vi "Autotrace.vi"() -> (2 "Center Position":dbl[](array[numeric])=[100.0, 100.0, 100.0], 3 "Final Count Rate":dbl format="%#.10g")   [LabVIEW 2020]
uses:
  Global Parameters.vi
  Global Parameter/NV Global.vi
  labview_control/LaoJi/NI CTR/NI DAQ Counter.lvlib
  Labview Library/Libraries/ASG8100CY/ASG8100CY.lvlib
panel:
  in  "Sample Rate (Hz)":dbl=50.0
  out "AutoTrace Data":dbl[][](array[numeric])
  in  "name":string="NV_1.17_"
  in  "save?":bool
  in  "Tab Control":T1(tab)
  in  "Stop":bool
  out "Start Point":dbl[](array[numeric])
  in  "Diameter xy":dbl=4.0
  in  "No. of Points":i32=50
  in  "move distance max":dbl=0.5
  in  "Diameter z":dbl=8.0
  out "X Indicator":bool
  out "Y Indicator":bool
  out "Z Indicator":bool
  out "Y":cluster{dbl[], "Best Gaussian Fit":dbl[]}[](graph)=[{[28.587433264887064, 28.667433264887062, 28.747433264887064, 28.827433264887063, 28.907433264887064, 28.987433264887063, 29.067433264887065, 29.147433264887063, 29.227433264887065, 29.307433264887063, 29.387433264887065, 29.467433264887063, 29.547433264887065, 29.627433264887063, 29.707433264887065, 29.787433264887063, 29.867433264887065, 29.947433264887064, 30.027433264887065, 30.107433264887064, 30.187433264887066, 30.267433264887064, 30.347433264887066, 30.427433264887064, 30.507433264887062, 30.587433264887064, 30.667433264887066, 30.747433264887064, 30.827433264887063, 30.907433264887064, 30.987433264887063, 31.067433264887065, 31.147433264887063, 31.227433264887065, 31.307433264887063, 31.387433264887065, 31.467433264887063, 31.547433264887065, 31.627433264887063, 31.707433264887065, 31.787433264887063, 31.867433264887065, 31.947433264887064, 32.027433264887065, 32.107433264887064, 32.18743326488706, 32.26743326488707, 32.347433264887066, 32.427433264887064, 32.50743326488706], "Best Gaussian Fit"=[82695.7939382761, 93035.93239563631, 104208.75707394363, 116210.11359683966, 129023.80448201254, 142620.50495842184, 156956.86080825518, 171974.8132803884, 187601.19363183164, 203747.62553370168, 220310.76741984417, 237172.9189336669, 254203.00610454116, 271257.94900932355, 288184.403780577, 304820.8583173002, 321000.0484018995, 336551.6486337933, 351305.1811783909, 365093.0753155868, 377753.80263689667, 389135.00690826605, 399096.5444274202, 407513.3503978308, 414278.0495345521, 419303.2347992863, 422523.34668930905, 423896.09660369105, 423403.39108770975, 421051.7287169694, 416872.0574510246, 410919.09683369054, 403270.14579218073, 394023.4123464537, 383295.9156795657, 371221.0232029976, 357945.6950340998, 343627.5153542803, 328431.5942305132, 312527.42458537646, 296085.7771505447, 279275.71161830187, 262261.775109772, 245201.44989429894, 228242.90147961042, 211523.06625001764, 195166.10528265772, 179282.23833600763, 163966.95976739613, 149300.62673344553]}, {[28.587433264887064, 28.667433264887062, 28.747433264887064, 28.827433264887063, 28.907433264887064, 28.987433264887063, 29.067433264887065, 29.147433264887063, 29.227433264887065, 29.307433264887063, 29.387433264887065, 29.467433264887063, 29.547433264887065, 29.627433264887063, 29.707433264887065, 29.787433264887063, 29.867433264887065, 29.947433264887064, 30.027433264887065, 30.107433264887064, 30.187433264887066, 30.267433264887064, 30.347433264887066, 30.427433264887064, 30.507433264887062, 30.587433264887064, 30.667433264887066, 30.747433264887064, 30.827433264887063, 30.907433264887064, 30.987433264887063, 31.067433264887065, 31.147433264887063, 31.227433264887065, 31.307433264887063, 31.387433264887065, 31.467433264887063, 31.547433264887065, 31.627433264887063, 31.707433264887065, 31.787433264887063, 31.867433264887065, 31.947433264887064, 32.027433264887065, 32.107433264887064, 32.18743326488706, 32.26743326488707, 32.347433264887066, 32.427433264887064, 32.50743326488706], "Best Gaussian Fit"=[0.0, 0.0, 0.0, 0.0, 0.0, 206291.54274517627, 210191.98673408732, 213652.8090545292, 210992.13509832733, 225995.6712662076, 229171.96204752172, 235716.96444444387, 260374.20344517086, 269183.87857142655, 282045.01726815425, 300870.52845503774, 336014.8514509855, 352432.5725864057, 368076.08672803076, 394901.02495494834, 414560.21447765, 432489.6705639836, 433552.6213811527, 438455.5715313964, 455299.529286137, 456372.0008292065, 459809.01578123606, 444017.0537733845, 438784.5826197389, 420773.64736858197, 379644.37848563184, 369423.66261220514, 344908.61083223054, 340345.2079602573, 322023.16098694917, 308115.01870457915, 290468.51555417373, 283489.69824613957, 283962.05635919375, 283721.7296458335, 283917.8453180592, 277165.3062343066, 272160.0475794274, 261937.72177790813, 260232.55700557673, 258499.65012753732, 247613.77779795573, 246263.40366328714, 240502.41945111495, 243778.22832663747]}]
  out "X":cluster{dbl[], "Best Gaussian Fit":dbl[]}[](graph)=[{[30.618585858585853, 30.69858585858585, 30.778585858585853, 30.85858585858585, 30.938585858585853, 31.01858585858585, 31.098585858585853, 31.17858585858585, 31.258585858585853, 31.33858585858585, 31.418585858585853, 31.49858585858585, 31.578585858585853, 31.65858585858585, 31.738585858585854, 31.818585858585852, 31.898585858585854, 31.978585858585852, 32.05858585858585, 32.138585858585856, 32.218585858585854, 32.29858585858585, 32.37858585858585, 32.458585858585856, 32.538585858585854, 32.61858585858585, 32.69858585858585, 32.778585858585856, 32.858585858585855, 32.93858585858585, 33.01858585858585, 33.09858585858585, 33.178585858585855, 33.25858585858585, 33.33858585858585, 33.41858585858585, 33.498585858585855, 33.57858585858585, 33.65858585858585, 33.73858585858585, 33.818585858585855, 33.898585858585854, 33.97858585858585, 34.05858585858585, 34.138585858585856, 34.218585858585854, 34.29858585858585, 34.37858585858585, 34.45858585858585, 34.538585858585854], "Best Gaussian Fit"=[199622.7652092626, 213700.13322189654, 227947.77524969875, 242271.18422272106, 256568.8961464526, 270733.556571258, 284653.1608456071, 298212.4509139653, 311294.44639794744, 323782.08305597847, 335559.92762615264, 346515.93468145275, 356543.20861001866, 365541.7322943554, 373420.0235902078, 380096.6813503637, 385501.7845142223, 389578.11066303233, 392282.1443552326, 393584.85039918293, 393472.1928493558, 391945.38675389026, 389020.87633961934, 384730.040182248, 379118.63075326587, 372245.9623411023, 364183.8675010448, 355015.44770309766, 344833.6485509264, 333739.6937011037, 321841.41431907495, 309251.5125047676, 296085.79758573393, 282461.43352867546, 268495.2340192452, 254302.03909833776, 239993.20374368748, 225675.2245959362, 211448.52631291925, 197406.42396979578, 183634.2726835259, 170208.81040218376, 157197.6947260679, 144659.22986625435, 132642.27552394307, 121186.32569384929, 110321.74223363581, 100070.12554876537, 90444.80294075941, 81451.41405397304]}, {[30.618585858585853, 30.69858585858585, 30.778585858585853, 30.85858585858585, 30.938585858585853, 31.01858585858585, 31.098585858585853, 31.17858585858585, 31.258585858585853, 31.33858585858585, 31.418585858585853, 31.49858585858585, 31.578585858585853, 31.65858585858585, 31.738585858585854, 31.818585858585852, 31.898585858585854, 31.978585858585852, 32.05858585858585, 32.138585858585856, 32.218585858585854, 32.29858585858585, 32.37858585858585, 32.458585858585856, 32.538585858585854, 32.61858585858585, 32.69858585858585, 32.778585858585856, 32.858585858585855, 32.93858585858585, 33.01858585858585, 33.09858585858585, 33.178585858585855, 33.25858585858585, 33.33858585858585, 33.41858585858585, 33.498585858585855, 33.57858585858585, 33.65858585858585, 33.73858585858585, 33.818585858585855, 33.898585858585854, 33.97858585858585, 34.05858585858585, 34.138585858585856, 34.218585858585854, 34.29858585858585, 34.37858585858585, 34.45858585858585, 34.538585858585854], "Best Gaussian Fit"=[0.0, 0.0, 0.0, 0.0, 0.0, 427244.8722271027, 437596.2068010136, 438557.34292178537, 447522.7808637517, 450272.5610295557, 462861.06273628754, 465668.3899037813, 460005.58720065054, 456337.9991536631, 449257.817837283, 448342.5759616434, 436186.2288725173, 430644.30916723004, 419807.75032678, 400558.9430741828, 384481.8022328452, 372598.71866850153, 355275.13386246277, 342864.4763392376, 318625.43663690117, 305968.09319236135, 295158.16662579577, 280150.94194027554, 263182.40619435295, 256594.04351134866, 253517.6315882785, 246929.03603153766, 242208.0360085657, 228934.00480565085, 225579.11596168345, 218747.91014951197, 215025.77963564653, 207010.84932462528, 210830.96445404616, 206259.81180164526, 204225.92522338819, 210423.6634213615, 203684.5686192836, 209968.62289134995, 204533.09352025428, 206559.33826787924, 203394.15591947164, 207928.7397448016, 205453.0602229333, 201667.86139781526]}]
  out "Z":cluster{dbl[], "Best Gaussian Fit":dbl[]}[](graph)=[{[47.76000000000001, 47.92000000000001, 48.08000000000001, 48.24000000000001, 48.40000000000001, 48.56000000000001, 48.72000000000001, 48.88000000000001, 49.04000000000001, 49.20000000000001, 49.360000000000014, 49.52000000000001, 49.680000000000014, 49.84000000000001, 50.000000000000014, 50.16000000000001, 50.320000000000014, 50.48000000000001, 50.640000000000015, 50.80000000000001, 50.960000000000015, 51.12000000000001, 51.280000000000015, 51.44000000000001, 51.60000000000001, 51.76000000000001, 51.920000000000016, 52.08000000000001, 52.24000000000001, 52.40000000000001, 52.56000000000001, 52.72000000000001, 52.88000000000001, 53.04000000000001, 53.20000000000001, 53.360000000000014, 53.52000000000001, 53.680000000000014, 53.84000000000001, 54.000000000000014, 54.16000000000001, 54.320000000000014, 54.48000000000001, 54.640000000000015, 54.80000000000001, 54.960000000000015, 55.12000000000001, 55.280000000000015, 55.44000000000001, 55.60000000000001], "Best Gaussian Fit"=[209099.73307391262, 218503.14461197148, 229355.6959593358, 241719.88156101448, 255620.83493327926, 271037.87859240867, 287896.9703361263, 306064.70466487855, 325344.52746696095, 345475.76446683565, 366135.9454640973, 386946.72907660797, 407483.5051154103, 427288.4889323076, 445886.84477118263, 462805.10789012676, 477590.94406552694, 489833.11476363277, 499180.42722509126, 505358.4545023384, 508182.9157852256, 507568.80692190514, 503534.6499186207, 496201.56499610166, 485787.2300702261, 472595.14800389623, 456999.9599731276, 439429.79620230943, 420346.82253882475, 400227.211264221, 379541.735522225, 358738.06678508525, 338225.66015664616, 318363.86532424996, 299453.6271605823, 281732.8651797201, 265375.36869575386, 250492.83345338725, 237139.50851200195, 225318.8254649993, 214991.345461141, 206083.37725441426, 198495.6818046096, 192111.77343650526, 186805.44102964734, 182447.23253688062, 178909.76143960972, 176071.79614687152, 173821.17726175574, 172056.67029302815]}, {[47.76000000000001, 47.92000000000001, 48.08000000000001, 48.24000000000001, 48.40000000000001, 48.56000000000001, 48.72000000000001, 48.88000000000001, 49.04000000000001, 49.20000000000001, 49.360000000000014, 49.52000000000001, 49.680000000000014, 49.84000000000001, 50.000000000000014, 50.16000000000001, 50.320000000000014, 50.48000000000001, 50.640000000000015, 50.80000000000001, 50.960000000000015, 51.12000000000001, 51.280000000000015, 51.44000000000001, 51.60000000000001, 51.76000000000001, 51.920000000000016, 52.08000000000001, 52.24000000000001, 52.40000000000001, 52.56000000000001, 52.72000000000001, 52.88000000000001, 53.04000000000001, 53.20000000000001, 53.360000000000014, 53.52000000000001, 53.680000000000014, 53.84000000000001, 54.000000000000014, 54.16000000000001, 54.320000000000014, 54.48000000000001, 54.640000000000015, 54.80000000000001, 54.960000000000015, 55.12000000000001, 55.280000000000015, 55.44000000000001, 55.60000000000001], "Best Gaussian Fit"=[0.0, 0.0, 0.0, 0.0, 0.0, 393271.00128946366, 407480.41678200994, 410814.7341749502, 426521.3026883778, 430066.65285827825, 443370.58597368945, 459367.2602933661, 461823.6110592089, 461604.39051720646, 457673.8141300071, 471897.3992822233, 475269.15246727964, 494259.5933463088, 489318.74382746057, 485038.7774016339, 492418.5246702464, 492340.1061251857, 496258.93171883747, 470118.45592524635, 447906.92402490036, 444693.88179068966, 425436.1282296754, 414968.0652258372, 401415.1316234149, 383381.7960970132, 371446.81388909504, 349417.72365313204, 332184.68010942376, 320808.8198801387, 312936.86398166575, 298427.2357123923, 292511.01335288194, 279437.24177576846, 273899.5635723089, 263004.1825411595, 257646.11261281034, 247225.51752630447, 245565.812568203, 241101.30046311184, 235636.8265278222, 232213.79944477836, 231398.6192754935, 224071.13931402928, 221070.99157966094, 218976.58246620942]}]
  out "Z Line Position":dbl[](array[numeric])=[-4.0, -3.84, -3.68, -3.52, -3.36, -3.2, -3.04, -2.88, -2.7199999999999998, -2.56, -2.4, -2.24, -2.08, -1.92, -1.7599999999999998, -1.6, -1.44, -1.2799999999999998, -1.12, -0.96, -0.7999999999999998, -0.6400000000000001, -0.48, -0.31999999999999984, -0.16000000000000014, 0.0, 0.16000000000000014, 0.3200000000000003, 0.4800000000000004, 0.6399999999999997, 0.7999999999999998, 0.96, 1.12, 1.2800000000000002, 1.4400000000000004, 1.6000000000000005, 1.7599999999999998, 1.92, 2.08, 2.24, 2.4000000000000004, 2.5600000000000005, 2.7199999999999998, 2.88, 3.04, 3.2, 3.3600000000000003, 3.5200000000000005, 3.6799999999999997, 3.84, 4.0]
  out "X Line Position":dbl[](array[numeric])=[-2.0, -1.92, -1.84, -1.76, -1.68, -1.6, -1.52, -1.44, -1.3599999999999999, -1.28, -1.2, -1.12, -1.04, -0.96, -0.8799999999999999, -0.8, -0.72, -0.6399999999999999, -0.56, -0.48, -0.3999999999999999, -0.32000000000000006, -0.24, -0.15999999999999992, -0.08000000000000007, 0.0, 0.08000000000000007, 0.16000000000000014, 0.2400000000000002, 0.31999999999999984, 0.3999999999999999, 0.48, 0.56, 0.6400000000000001, 0.7200000000000002, 0.8000000000000003, 0.8799999999999999, 0.96, 1.04, 1.12, 1.2000000000000002, 1.2800000000000002, 1.3599999999999999, 1.44, 1.52, 1.6, 1.6800000000000002, 1.7600000000000002, 1.8399999999999999, 1.92, 2.0]
  out "Y line Position":dbl[](array[numeric])=[-2.0, -1.92, -1.84, -1.76, -1.68, -1.6, -1.52, -1.44, -1.3599999999999999, -1.28, -1.2, -1.12, -1.04, -0.96, -0.8799999999999999, -0.8, -0.72, -0.6399999999999999, -0.56, -0.48, -0.3999999999999999, -0.32000000000000006, -0.24, -0.15999999999999992, -0.08000000000000007, 0.0, 0.08000000000000007, 0.16000000000000014, 0.2400000000000002, 0.31999999999999984, 0.3999999999999999, 0.48, 0.56, 0.6400000000000001, 0.7200000000000002, 0.8000000000000003, 0.8799999999999999, 0.96, 1.04, 1.12, 1.2000000000000002, 1.2800000000000002, 1.3599999999999999, 1.44, 1.52, 1.6, 1.6800000000000002, 1.7600000000000002, 1.8399999999999999, 1.92, 2.0]
  in  "Limit":T2={"width threshold -"=0.05, "width threshold +"=6.0, "counts threshold"=15000.0}
  out "NV or not?":bool
  out "Laser On":bool=TRUE
  out "Positioner\nerror":errorcluster
  in  "AutoTrace \nData base path":path=path "I:/AutoTrace"
  # "Counter Settings"
  # "Clock Settings"
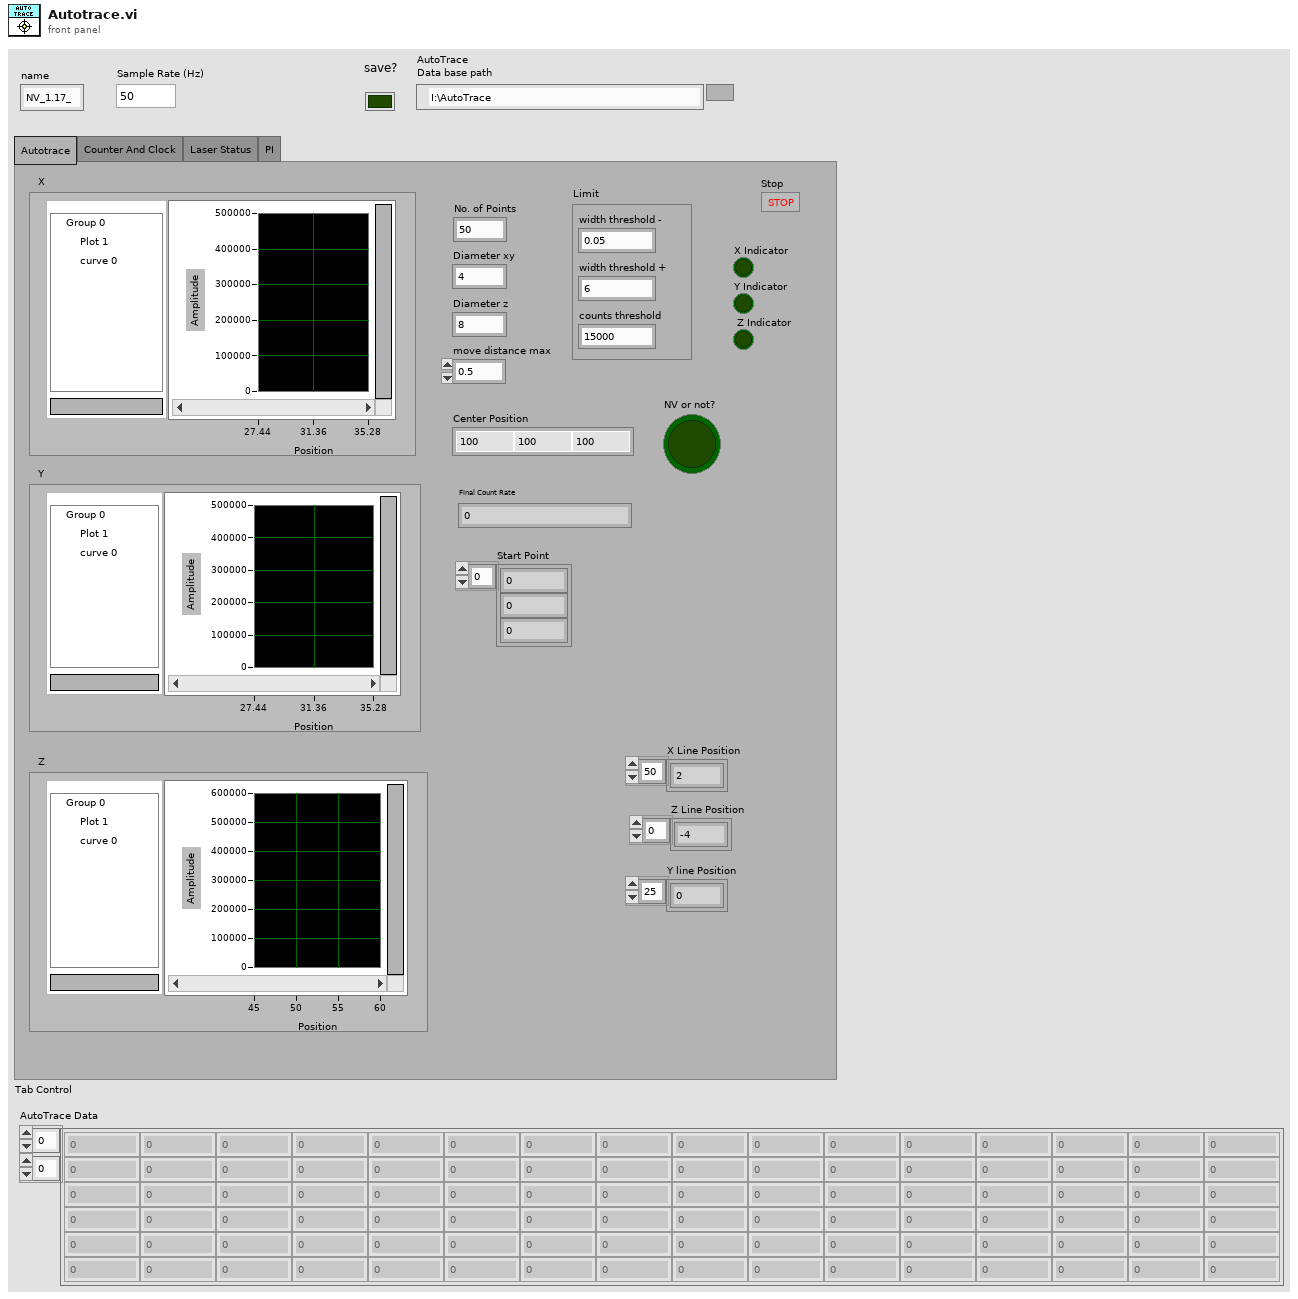
[diagram p1: front panel]
types:
  T1 = enum32{"Autotrace", "Counter And Clock", "Laser Status", "PI"}
  T2 = cluster{"width threshold -":dbl, "width threshold +":dbl, "counts threshold":dbl}
  T3 = typedef "imagedata.ctl" = cluster{"image type":i32, "image depth":i32, "image":u8[], "mask":u8[], "colors":u32[], "Rectangle":cluster{"left":i16, "top":i16, "right":i16, "bottom":i16}}
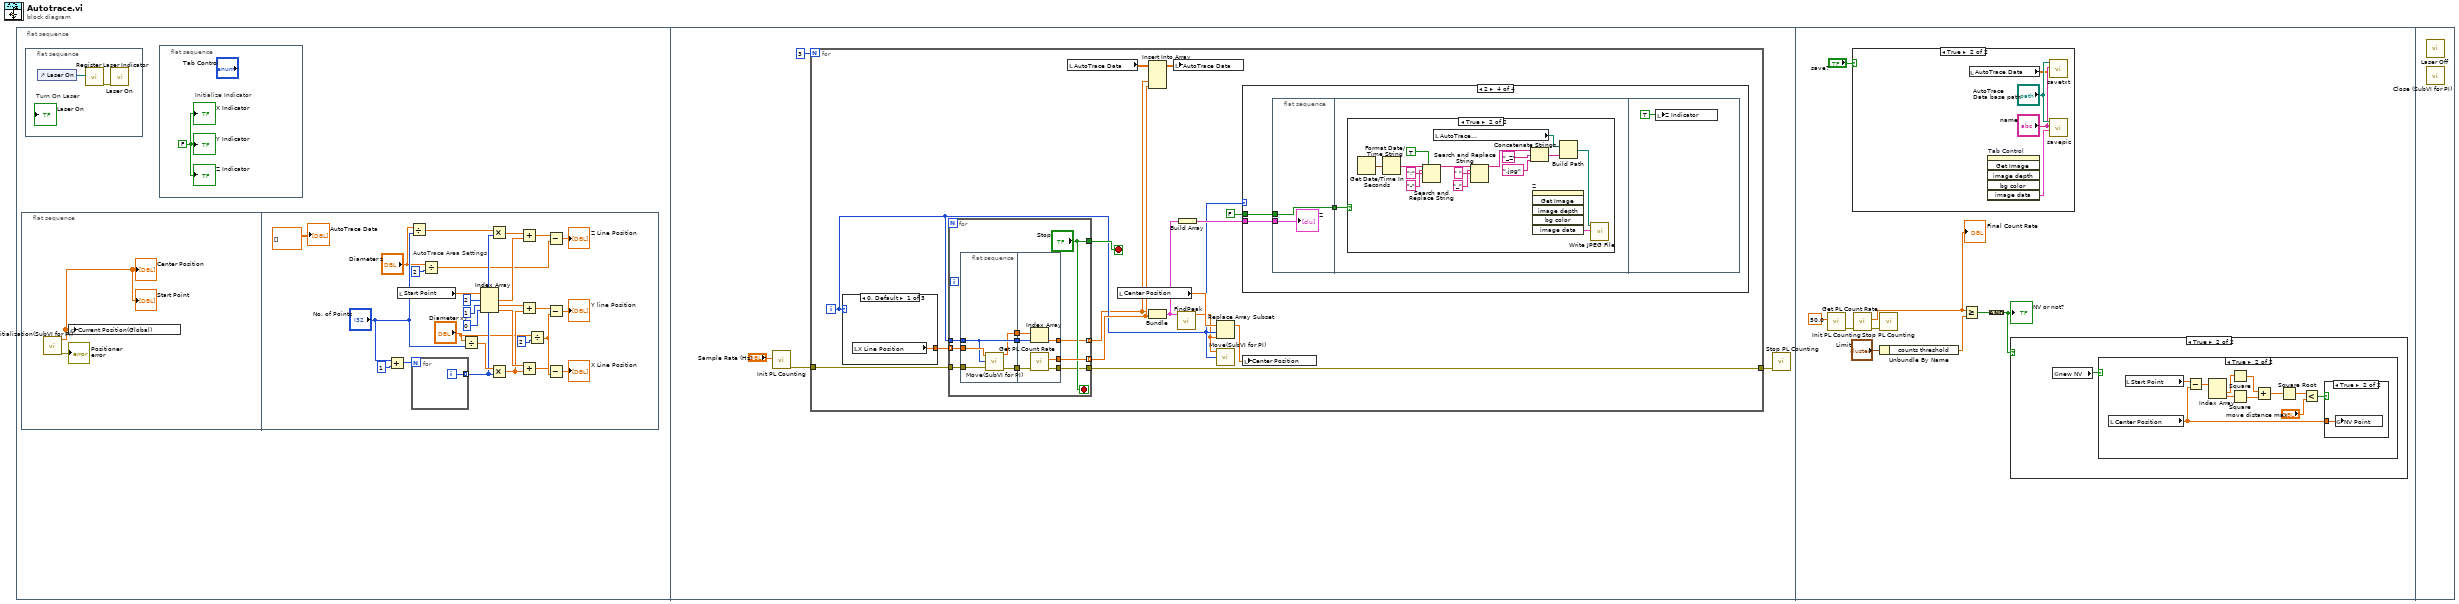
[diagram p0: block diagram]
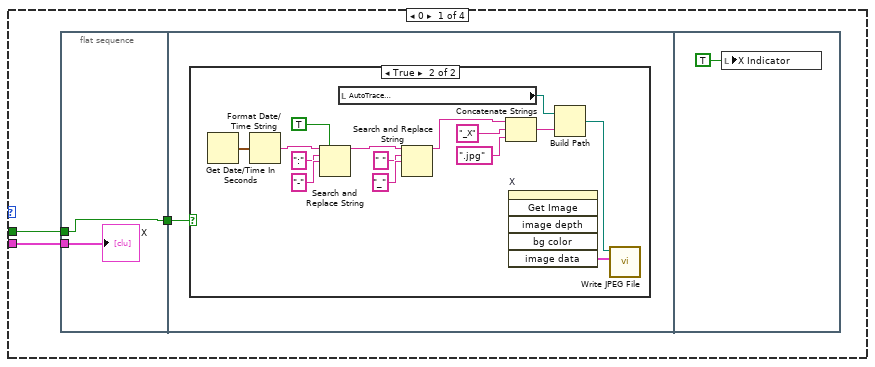
[diagram p2: hidden frame]
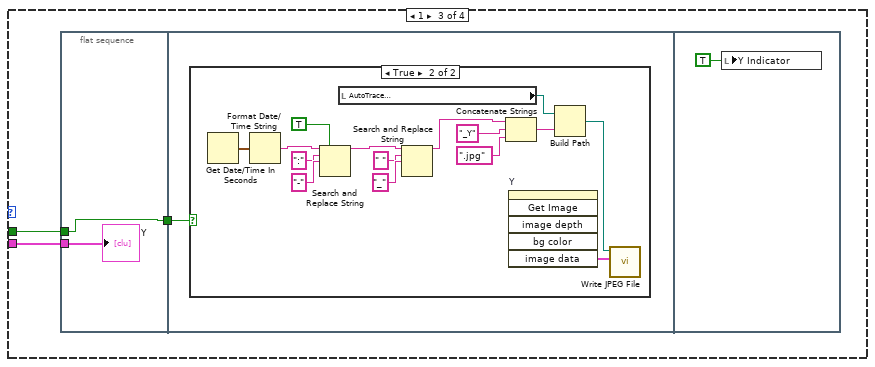
[diagram p5: hidden frame]
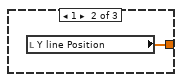
[diagram p8: hidden frame]
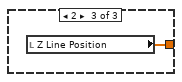
[diagram p9: hidden frame]
diagram:
  n1 = flat-sequence {
    frame #0 {
      n2 = flat-sequence {
        frame #0 {
          n3 = call "Initialization(SubVI for PI).vi"() -> ("error out"=→"Positioner\nerror":errorcluster, "Position"=w4:dbl[])  [unwired: 10 in]
          "Start Point" <- w4
          "Center Position" <- w4
          n4 = global write "Global Parameters.vi" "Current Position(Global)"(w4) -> ()
        }
        frame #1 {
          # "AutoTrace Area Settings"
          n5 = Add(x="No. of Points", y=1) -> (x+y=w32:i32)
          n6 = local read "Start Point"() -> (w24:dbl[])
          n7 = Divide(x="Diameter z", y="No. of Points") -> (x/y=w28:dbl)
          n8 = for {
            N: w32 -> [_]
            tunnel: [w34] -> w29 mode=indexing
            i -> [w34]
          }
          n9 = Divide(x="Diameter z", y=2) -> (x/y=w16:dbl)
          n10 = Divide(x="Diameter xy", y="No. of Points") -> (x/y=w30:dbl)
          n11 = Index Array(array=w24, index #1=2, index #2=1, index #3=0) -> (element #1=w23:dbl, element #2=w21:dbl, element #3=w20:dbl)
          n12 = Multiply(x=w28, y=w29) -> (x*y=w22:dbl[])
          n13 = Multiply(x=w30, y=w29) -> (x*y=w19:dbl[])
          n14 = Add(x=w22, y=w23) -> (x+y=w18:dbl[])
          n15 = Add(x=w21, y=w19) -> (x+y=w11:dbl[])
          n16 = Add(x=w20, y=w19) -> (x+y=w8:dbl[])
          n17 = Divide(x="Diameter xy", y=2) -> (x/y=w9:dbl)
          n18 = Subtract(x=w18, y=w16) -> (x-y=→"Z Line Position":dbl[])
          n19 = Subtract(x=w11, y=w9) -> (x-y=→"Y line Position":dbl[])
          n20 = Subtract(x=w8, y=w9) -> (x-y=→"X Line Position":dbl[])
          "AutoTrace Data" <- dbl[][] [] ("AutoTrace Data")
        }
      }
      n21 = flat-sequence {
        frame #0 {
          # "Turn On Laser"
          n22 = control-ref of="Laser On"() -> (w3:refnum<vi>)
          n23 = call "Register Laser Indicator.vi"("Laser Indicator Ref"=w3) -> ("error out"=w2:errorcluster)  [unwired: 10 in]
          n24 = call "Laser On.vi"("error in"=w2) -> ()  [unwired: 10 in, 1 out]
        }
      }
      n25 = flat-sequence {
        frame #0 {
          w1 = FALSE
          # "Initialize Indicator"
          "X Indicator" <- w1
          "Y Indicator" <- w1
          "Z Indicator" <- w1
        }
      }
    }
    frame #1 {
      n26 = call "Init PL Counting.vi"("Sample Rate (Hz)"="Sample Rate (Hz)") -> ("error out"=w36:errorcluster)  [unwired: 10 in]
      n27 = for {
        N: 3 -> [_]
        tunnel: w36 -> [w44]
        tunnel: [w43] -> w35
        i -> [w42]
        stop <- w51 stop-if-true
        n28 = case shown="0, Default" w42 {
          tunnel: [w120 w121 w122] -> w40
          frame 0, Default {
            n29 = local read "X Line Position"() -> (w120:dbl[])
          }
          frame 1 {
            n30 = local read "Y line Position"() -> (w121:dbl[])
          }
          frame 2 {
            n31 = local read "Z Line Position"() -> (w122:dbl[])
          }
        }
        n32 = for {
          tunnel: w40 -> [w132] mode=indexing
          tunnel: w42 -> [w131]
          tunnel: [w130] -> w46 mode=indexing
          tunnel: ["Stop"] -> w51
          tunnel: w44 -> [w128]
          tunnel: [w126] -> w43
          tunnel: [w123] -> w39 mode=indexing
          stop <- "Stop" stop-if-true
          n33 = flat-sequence {
            tunnel: w132 -> [w137]
            tunnel: w131 -> [w134]
            tunnel: w128 -> [w136]
            tunnel: [w135] -> w127
            tunnel: [w134] -> w125
            tunnel: [w133] -> w124
            tunnel: [w143] -> w130
            tunnel: w127 -> [w142]
            tunnel: [w141] -> w126
            tunnel: w125 -> [w140]
            tunnel: w124 -> [w139]
            tunnel: [w138] -> w123
            frame #0 {
              n34 = call "Move(SubVI for PI).vi"("Goal"=w137, "index"=w134, "error in"=w136) -> ("Position After Move"=w133:dbl[], "error out"=w135:errorcluster)  [unwired: 3 in]
            }
            frame #1 {
              n35 = Index Array(array=w139, index=w140) -> (element=w138:dbl)
              n36 = call "Get PL Count Rate.vi"("error in (no error)"=w142) -> ("error out"=w141:errorcluster, "Count Rate"=w143:dbl)  [unwired: 8 in, 1 out]
            }
          }
        }
        n37 = local read "AutoTrace Data"() -> (w47:dbl[][])
        n38 = local read "Center Position"() -> (w50:dbl[])
        n39 = Insert Into Array(array=w47, new element #1=w39, new element #2=w46) -> (w48:dbl[][])  [unwired: 2 in]
        n40 = Bundle(w39, w46) -> (w45:cluster{dbl[], dbl[]})  [unwired: 1 in]
        n41 = local write "AutoTrace Data"(w48) -> ()
        n42 = call "FindPeak.vi"("Input XY"=w45) -> ("Peak Position"=w41:dbl)  [unwired: 8 in, 2 out]
        n43 = Build Array(w45) -> (w53:cluster{dbl[], dbl[]}[])
        n44 = Replace Array Subset(array=w50, new element=w41, index=w42) -> (w49:dbl[])
        n45 = call "Move(SubVI for PI).vi"("Goal"=w41, "index"=w42) -> ()  [unwired: 4 in, 2 out]
        n46 = case shown="2" w42 {
          tunnel: w53 -> [w56 _ w78 w100]
          tunnel: FALSE -> [w54 _ w77 w98]
          frame 0 {
            n47 = flat-sequence {
              tunnel: w56 -> [w58]
              tunnel: [w57] -> w55
              tunnel: w54 -> [w57]
              tunnel: w55 -> [w59]
              frame #0 {
                "X" <- w58
              }
              frame #1 {
                n48 = case shown="True" w59 {
                  frame False {
                  }
                  frame True {
                    n49 = Get Date/Time In Seconds() -> (seconds since 1Jan1904=w74:timestamp)
                    n50 = Format Date/Time String(seconds (now)=w74) -> (date/time string=w67:string)  [unwired: 2 out]
                    n51 = Search and Replace String(replace all?=TRUE ("replace all? (F)"), input string=w67, search string=":", replace string="-" ("replace string (\"\")")) -> (result string=w71:string)  [unwired: 1 in, 6 out]
                    n52 = local read "AutoTrace \nData base path"() -> (w60:path)
                    n53 = Search and Replace String(input string=w71, search string=" ", replace string="_" ("replace string (\"\")")) -> (result string=w64:string)  [unwired: 1 in, 7 out]
                    n54 = Concatenate Strings(w64, "_X" ("string"), ".jpg" ("string")) -> (w66:string)
                    n55 = invoke on="X" class="MixedGraph (严格)" method="Get Image"() -> ("image data"=w61:T3)  [unwired: 6 in, 5 out]
                    n56 = Build Path(base path=w60, name or relative path=w66) -> (appended path=w65:path)
                    n57 = call <vilib>:"Write JPEG File.vi"("image data"=w61, "path to JPEG file"=w65) -> ()  [unwired: 1 in, 9 out]
                  }
                }
              }
              frame #2 {
                n58 = local write "X Indicator"(TRUE) -> ()
              }
            }
          }
          frame 3, Default {
          }
          frame 1 {
            n59 = flat-sequence {
              tunnel: w78 -> [w80]
              tunnel: w77 -> [w79]
              tunnel: [w79] -> w76
              tunnel: w76 -> [w81]
              frame #0 {
                "Y" <- w80
              }
              frame #1 {
                n60 = case shown="True" w81 {
                  frame False {
                  }
                  frame True {
                    n61 = Get Date/Time In Seconds() -> (seconds since 1Jan1904=w96:timestamp)
                    n62 = Format Date/Time String(seconds (now)=w96) -> (date/time string=w89:string)  [unwired: 2 out]
                    n63 = Search and Replace String(replace all?=TRUE ("replace all? (F)"), input string=w89, search string=":", replace string="-" ("replace string (\"\")")) -> (result string=w93:string)  [unwired: 1 in, 6 out]
                    n64 = local read "AutoTrace \nData base path"() -> (w86:path)
                    n65 = Search and Replace String(input string=w93, search string=" ", replace string="_" ("replace string (\"\")")) -> (result string=w85:string)  [unwired: 1 in, 7 out]
                    n66 = Concatenate Strings(w85, "_Y" ("string"), ".jpg" ("string")) -> (w88:string)
                    n67 = invoke on="Y" class="MixedGraph (严格)" method="Get Image"() -> ("image data"=w82:T3)  [unwired: 6 in, 5 out]
                    n68 = Build Path(base path=w86, name or relative path=w88) -> (appended path=w87:path)
                    n69 = call <vilib>:"Write JPEG File.vi"("image data"=w82, "path to JPEG file"=w87) -> ()  [unwired: 1 in, 9 out]
                  }
                }
              }
              frame #2 {
                n70 = local write "Y Indicator"(TRUE) -> ()
              }
            }
          }
          frame 2 {
            n71 = flat-sequence {
              tunnel: w100 -> [w102]
              tunnel: [w101] -> w99
              tunnel: w98 -> [w101]
              tunnel: w99 -> [w103]
              frame #0 {
                "Z" <- w102
              }
              frame #1 {
                n72 = case shown="True" w103 {
                  frame False {
                  }
                  frame True {
                    n73 = Get Date/Time In Seconds() -> (seconds since 1Jan1904=w118:timestamp)
                    n74 = Format Date/Time String(seconds (now)=w118) -> (date/time string=w111:string)  [unwired: 2 out]
                    n75 = Search and Replace String(replace all?=TRUE ("replace all? (F)"), input string=w111, search string=":", replace string="-" ("replace string (\"\")")) -> (result string=w115:string)  [unwired: 1 in, 6 out]
                    n76 = local read "AutoTrace \nData base path"() -> (w108:path)
                    n77 = Search and Replace String(input string=w115, search string=" ", replace string="_" ("replace string (\"\")")) -> (result string=w107:string)  [unwired: 1 in, 7 out]
                    n78 = Concatenate Strings(w107, "_Z" ("string"), ".jpg" ("string")) -> (w110:string)
                    n79 = invoke on="Z" class="MixedGraph (严格)" method="Get Image"() -> ("image data"=w104:T3)  [unwired: 6 in, 5 out]
                    n80 = Build Path(base path=w108, name or relative path=w110) -> (appended path=w109:path)
                    n81 = call <vilib>:"Write JPEG File.vi"("image data"=w104, "path to JPEG file"=w109) -> ()  [unwired: 1 in, 9 out]
                  }
                }
              }
              frame #2 {
                n82 = local write "Z Indicator"(TRUE) -> ()
              }
            }
          }
        }
        n83 = local write "Center Position"(w49) -> ()
      }
      n84 = call "Stop PL Counting.vi"("error in (no error)"=w35) -> ()  [unwired: 10 in, 1 out]
    }
    frame #2 {
      n85 = call "Init PL Counting.vi"("Sample Rate (Hz)"=50.0) -> ("error out"=w147:errorcluster)  [unwired: 10 in]
      n86 = case shown="True" "save?" {
        frame False {
        }
        frame True {
          n87 = local read "AutoTrace Data"() -> (w167:dbl[][])
          n88 = invoke on="Tab Control" class="TabCtl (strict)" method="Get Image"() -> ("image data"=w166:T3)  [unwired: 6 in, 5 out]
          n89 = call "savetxt.vi"("2D data"=w167, "name"="name", "path"="AutoTrace \nData base path") -> ()  [unwired: 8 in, 1 out]
          n90 = call "savepic.vi"("image data"=w166, "name"="name", "Path"="AutoTrace \nData base path") -> ()  [unwired: 7 in, 2 out]
        }
      }
      n91 = call "Get PL Count Rate.vi"("error in (no error)"=w147) -> ("error out"=w146:errorcluster, "Count Rate"=w145:dbl)  [unwired: 8 in, 1 out]
      "Final Count Rate" <- w145
      n92 = call "Stop PL Counting.vi"("error in (no error)"=w146) -> ()  [unwired: 10 in, 1 out]
      n93 = Unbundle By Name("Limit") -> ("counts threshold"=w151:dbl)
      n94 = Greater Or Equal?(x=w145, y=w151) -> (x >= y?=w152:bool)
      n95 = Compound Arithmetic op=AND(w152) -> (w148:bool)
      "NV or not?" <- w148
      n96 = case shown="True" w148 {
        frame False {
        }
        frame True {
          n97 = global read "NV Global.vi" "new NV"() -> (w153:bool)
          n98 = case shown="True" w153 {
            frame False {
            }
            frame True {
              n99 = local read "Center Position"() -> (w154:dbl[])
              n100 = local read "Start Point"() -> (w157:dbl[])
              n101 = Subtract(x=w157, y=w154) -> (x-y=w164:dbl[])
              n102 = Index Array(array=w164) -> (element #1=w163:dbl, element #2=w162:dbl)  [unwired: 2 in]
              n103 = Square(x=w163) -> (x^2=w161:dbl)
              n104 = Square(x=w162) -> (x^2=w160:dbl)
              n105 = Add(x=w161, y=w160) -> (x+y=w159:dbl)
              n106 = Square Root(x=w159) -> (sqrt(x)=w158:dbl)
              n107 = Less?(x=w158, y="move distance max") -> (x < y?=w155:bool)
              n108 = case shown="True" w155 {
                tunnel: w154 -> [_ w165]
                frame False {
                }
                frame True {
                  n109 = global write "NV Global.vi" "NV Point"(w165) -> ()
                }
              }
            }
          }
        }
      }
    }
    frame #3 {
      n110 = call "Laser Off.vi"() -> ()  [unwired: 11 in, 1 out]
      n111 = call "Close (SubVI for PI).vi"() -> ()  [unwired: 12 in]
    }
  }
